vi "刷新表格.vi"(8 "列":i32, 9 "行":i32, 11 "引用in":refnum<vi>) -> (3 "引用out":refnum<vi>)   [LabVIEW 2011]
uses:
  <vilib>/Utility/miscctls.llb/LVRowAndColumnTypeDef.ctl
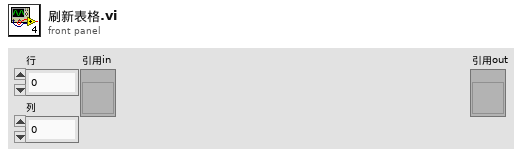
[diagram p1: front panel]
types:
  T1 = typedef "LVRowAndColumnTypeDef.ctl" = cluster{"Row":i32, "Column":i32}
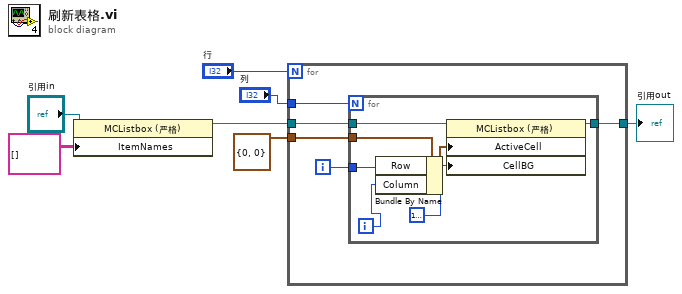
[diagram p0: block diagram]
diagram:
  n1 = property class="MCListbox (严格)"(reference="引用in", "ItemNames"=string[][] [] ("项名")) -> (reference out=w7:refnum<vi>)  [unwired: 1 in, 1 out]
  n2 = for {
    N: "行" -> [_]
    tunnel: w7 -> [w12]
    tunnel: T1 {"Row"=0, "Column"=0} ("活动单元格:活动单元格") -> [w11]
    tunnel: [w9] -> w2
    tunnel: "列" -> [w8]
    i -> [w10]
    n3 = for {
      N: w8 -> [_]
      tunnel: w12 -> [w19]
      tunnel: w11 -> [w18]
      tunnel: w10 -> [w16]
      tunnel: [w14] -> w9
      i -> [w15]
      n4 = Bundle By Name(cluster=w18, "Row"=w16, "Column"=w15) -> (w17:T1)
      n5 = property class="MCListbox (严格)"(reference=w19, "ActiveCell"=w17, "CellBG"=u32 16777238) -> (reference out=w14:refnum<vi>)  [unwired: 1 in, 1 out]
    }
  }
  "引用out" <- w2
